vi "Read Thermocouples.vi"(8 "error in (no error)":errorcluster, 10 "Thermocouple Count (15)":i32=15) -> (0 "error out":errorcluster, 2 "Temperatures (C)":dbl[](array[numeric]))   [LabVIEW 2019]
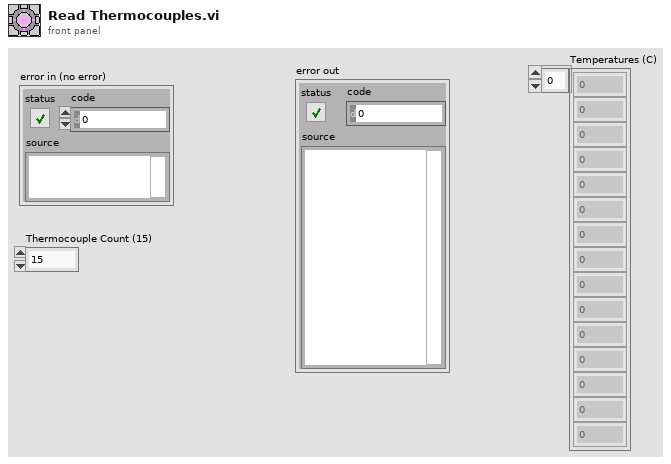
[diagram p1: front panel]
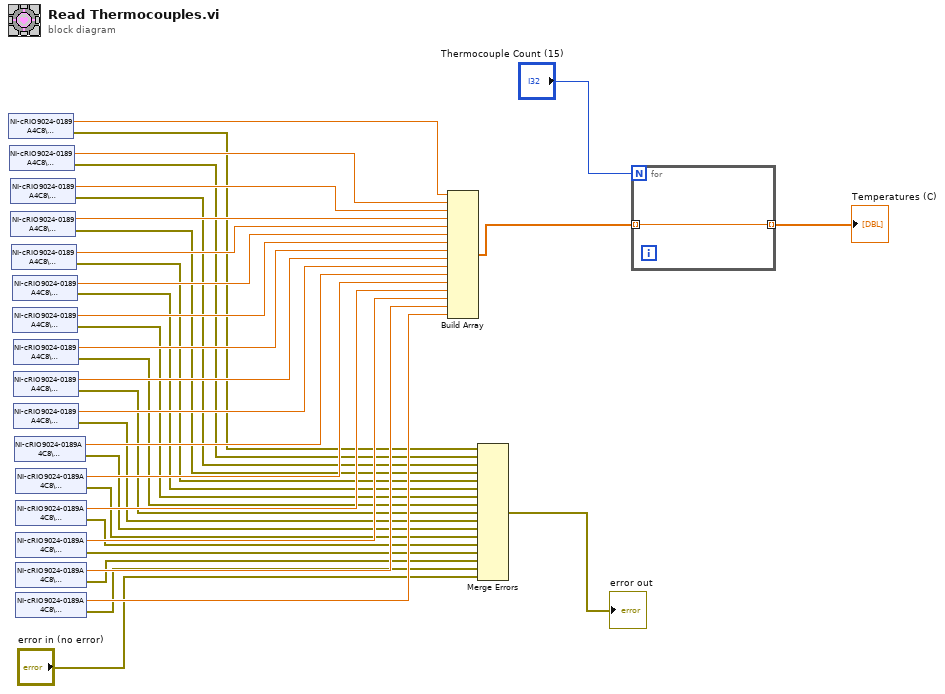
[diagram p0: block diagram]
diagram:
  n1 = shared-variable "NI-cRIO9024-0189A4C8\\Thermocouples\\TC0"() -> (w37:dbl, error out=w6:errorcluster)  [unwired: 1 in]
  n2 = shared-variable "NI-cRIO9024-0189A4C8\\Thermocouples\\TC1"() -> (w36:dbl, error out=w7:errorcluster)  [unwired: 1 in]
  n3 = shared-variable "NI-cRIO9024-0189A4C8\\Thermocouples\\TC2"() -> (w35:dbl, error out=w8:errorcluster)  [unwired: 1 in]
  n4 = shared-variable "NI-cRIO9024-0189A4C8\\Thermocouples\\TC3"() -> (w34:dbl, error out=w9:errorcluster)  [unwired: 1 in]
  n5 = shared-variable "NI-cRIO9024-0189A4C8\\Thermocouples\\TC4"() -> (w33:dbl, error out=w10:errorcluster)  [unwired: 1 in]
  n6 = shared-variable "NI-cRIO9024-0189A4C8\\Thermocouples\\TC5"() -> (w32:dbl, error out=w11:errorcluster)  [unwired: 1 in]
  n7 = shared-variable "NI-cRIO9024-0189A4C8\\Thermocouples\\TC6"() -> (w31:dbl, error out=w12:errorcluster)  [unwired: 1 in]
  n8 = shared-variable "NI-cRIO9024-0189A4C8\\Thermocouples\\TC7"() -> (w30:dbl, error out=w13:errorcluster)  [unwired: 1 in]
  n9 = shared-variable "NI-cRIO9024-0189A4C8\\Thermocouples\\TC8"() -> (w29:dbl, error out=w14:errorcluster)  [unwired: 1 in]
  n10 = shared-variable "NI-cRIO9024-0189A4C8\\Thermocouples\\TC9"() -> (w28:dbl, error out=w15:errorcluster)  [unwired: 1 in]
  n11 = shared-variable "NI-cRIO9024-0189A4C8\\Thermocouples\\TC10"() -> (w27:dbl, error out=w16:errorcluster)  [unwired: 1 in]
  n12 = shared-variable "NI-cRIO9024-0189A4C8\\Thermocouples\\TC11"() -> (w26:dbl, error out=w17:errorcluster)  [unwired: 1 in]
  n13 = shared-variable "NI-cRIO9024-0189A4C8\\Thermocouples\\TC12"() -> (w25:dbl, error out=w18:errorcluster)  [unwired: 1 in]
  n14 = shared-variable "NI-cRIO9024-0189A4C8\\Thermocouples\\TC13"() -> (w24:dbl, error out=w19:errorcluster)  [unwired: 1 in]
  n15 = shared-variable "NI-cRIO9024-0189A4C8\\Thermocouples\\TC14"() -> (w23:dbl, error out=w20:errorcluster)  [unwired: 1 in]
  n16 = shared-variable "NI-cRIO9024-0189A4C8\\Thermocouples\\TC15"() -> (w22:dbl, error out=w21:errorcluster)  [unwired: 1 in]
  n17 = Build Array(w37, w36, w35, w34, w33, w32, w31, w30, w29, w28, w27, w26, w25, w24, w23, w22) -> (w3:dbl[])
  n18 = Merge Errors(w6, w7, w8, w9, w10, w11, w12, w13, w14, w15, w16, w17, w18, w19, w20, w21, "error in (no error)") -> (→"error out":errorcluster)
  n19 = for {
    N: "Thermocouple Count (15)" -> [_]
    tunnel: w3 -> [w38] mode=indexing
    tunnel: [w38] -> w1 mode=indexing
  }
  "Temperatures (C)" <- w1
